vi "iFlex - Set Max.vi"() -> (3 "iFlex Enabled":bool)   [LabVIEW 2020]
uses:
  Thorlabs/LSM_SDK/ThorConfocal.lvlib
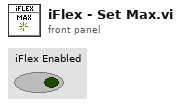
[diagram p1: front panel]
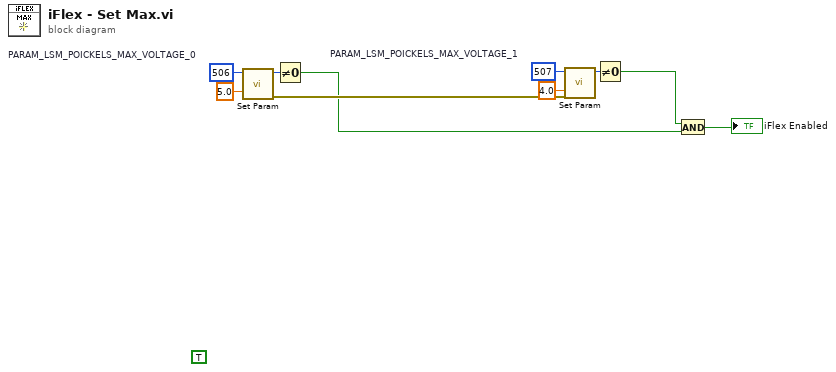
[diagram p0: block diagram]
diagram:
  w9 = 507  # PARAM_LSM_POICKELS_MAX_VOLTAGE_1
  w7 = 506  # PARAM_LSM_POICKELS_MAX_VOLTAGE_0
  (unwired) TRUE
  n1 = call "Set Param.vi"("param"=5.0, "paramID"=w7) -> ("error out"=w6:errorcluster, "function return"=w5:i32)  [unwired: 4 in]
  n2 = Not Equal To 0?(x=w5) -> (x != 0?=w2:bool)
  n3 = call "Set Param.vi"("error in (no error)"=w6, "param"=4.0, "paramID"=w9) -> ("function return"=w4:i32)  [unwired: 3 in, 1 out]
  n4 = Not Equal To 0?(x=w4) -> (x != 0?=w3:bool)
  n5 = And(x=w3, y=w2) -> (x .and. y?=→"iFlex Enabled":bool)
